vi "Stage Motor Test.vi"() -> ()   [LabVIEW 2016]
uses:
  <vilib>/Platform/TimedLoop/XDataNode/timing_clust.ctl
  <vilib>/Platform/TimedLoop/XDataNode/nitl_modes.ctl
  <vilib>/Platform/TimedLoop/XDataNode/wakeup.ctl
  <vilib>/DAQmx/write.llb/DAQmx Write (Analog 1D DBL NChan 1Samp).vi
  <vilib>/FPGAPlugInAG/PXI-7833R/niLvFpga_Open_PXI-7833R.vi
  <vilib>/Utility/error.llb/Error Cluster From Error Code.vi
  <vilib>/rvi/errors/niLvFpgaAdjustHostInterfaceError.vi
  <vilib>/DAQmx/create/channels.llb/DAQmx Create Channel (AO-Voltage-Basic).vi
  <vilib>/DAQmx/miscellaneous.llb/DAQmx Fill In Error Info.vi
  <vilib>/FPGAPlugInAG/PXI-7833R/niLvFpga_Reset_PXI-7833R.vi
  <vilib>/FPGAPlugInAG/PXI-7833R/niLvFpga_Close_PXI-7833R.vi
  <vilib>/Platform/TimedLoop/XDataNode/XDataNode.xnode
  <vilib>/rvi/interface/nirviOpenFPGA/nirviOpenFPGA.xnode
  FPGA Bitfiles/PhantomControlPI_FPGATarget_QuadCtr2_E2412E44.lvbitx
  IRISS_FPGA_IO.vi
  <vilib>/rvi/interface/nirviReadWriteControl/nirviReadWriteControl.xnode
  <vilib>/rvi/interface/nirviMethod/nirviMethod.xnode
  <vilib>/rvi/interface/nirviCloseFPGA/nirviCloseFPGA.xnode
  <vilib>/Platform/TimedLoop/XDataNode/XDNodeRunTimeDep.lvlib
  NiFpgaLv.dll
panel:
  out "Waveform Chart":T1(graph)
  out "Error(s) Out on Program End":errorcluster
  in  "Stage PID Cluster":T2={"Stage Z PID"={"Kp"=0.0005, "Kd"=0.001, "Ki"=0.0}, "Stage Y PID"={"Kp"=0.0003, "Kd"=0.01, "Ki"=0.0}, "Stage X PID"={"Kp"=0.0003, "Kd"=0.01, "Ki"=0.0}}
  in  "Stage cmd Posit [mm]":dbl[](array[numeric])=[12.0, 0.0, 0.0] min=0.0 max=12.0 step=0.1
  out "Stage out Posit [mm]":dbl[](array[numeric])=[12.0, 0.0, 0.0]
  in  "stop":bool
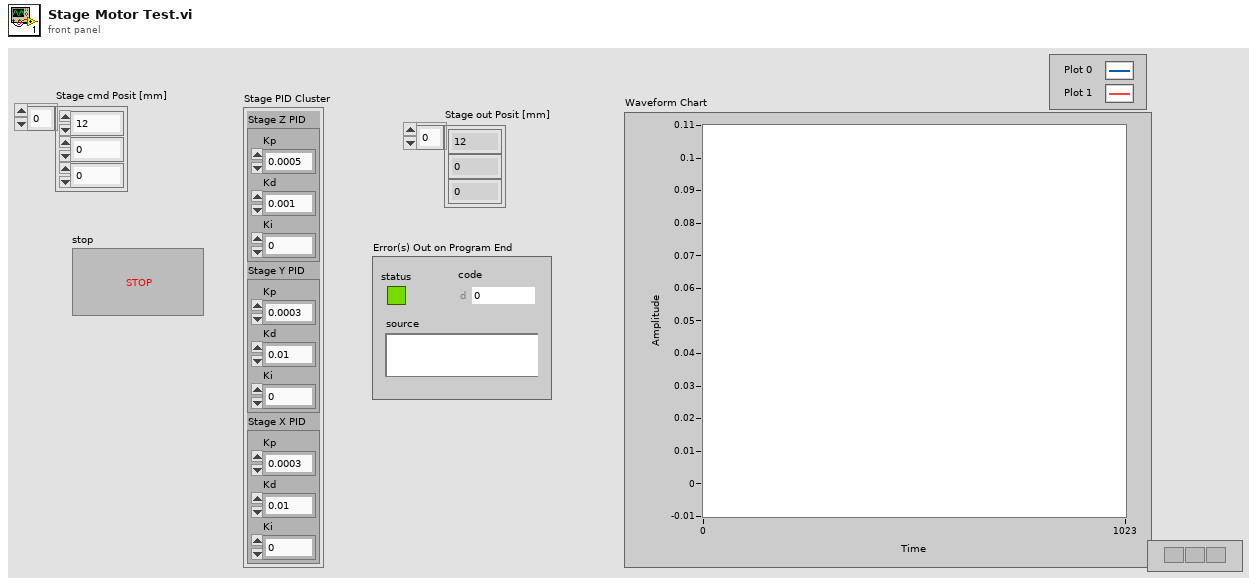
[diagram p1: front panel]
types:
  T1 = cluster{"StagePosition - X":dbl, "StagePosition - X":dbl}
  T2 = cluster{"Stage Z PID":cluster{"Kp":dbl, "Kd":dbl, "Ki":dbl}, "Stage Y PID":cluster{"Kp":dbl, "Kd":dbl, "Ki":dbl}, "Stage X PID":cluster{"Kp":dbl, "Kd":dbl, "Ki":dbl}}
  T3 = typedef "XDNodeRunTimeDep.lvlib/timing_clust.ctl" = cluster{"Expected End [f-1]":u64, "Actual End [f-1]":u64, "Finished Late? [f-1]":bool, "Expected End [i-1]":u64, "Actual End [i-1]":u64, "Finished Late? [i-1]":bool, "Expected Start [i]":u64, "Actual Start [i]":u64, "Expected Start [f]":u64, "Actual Start [f]":u64, "Source Name":string, "Structure Name":string, "Period":i64, "Deadline":i64, "Offset":i64, "Start":i64, "Priority":i32, "Timeout":i32, "Mode":T4, "Wakeup Reason":T5, "Error":errorcluster, "Source Type":string, "Secondary Source Type":string, "Global End Time":u64, "Global Start Time":u64, "Frame Duration":u64, "Iteration Duration":u64, "Assigned CPU":i32, "I/O Scan Engine Mode":u32}
  T4 = typedef "XDNodeRunTimeDep.lvlib/nitl_modes.ctl" = enum32{"No Change", "Process missed periods, maintain original phase", "Discard missed periods, maintain original phase", "Process missed periods, ignore original phase", "Discard missed periods, ignore original phase"}
  T5 = typedef "XDNodeRunTimeDep.lvlib/wakeup.ctl" = enum32{"Normal", "Aborted", "Asynchronous wakeup", "Timing source error", "Timed loop error", "Timeout"}
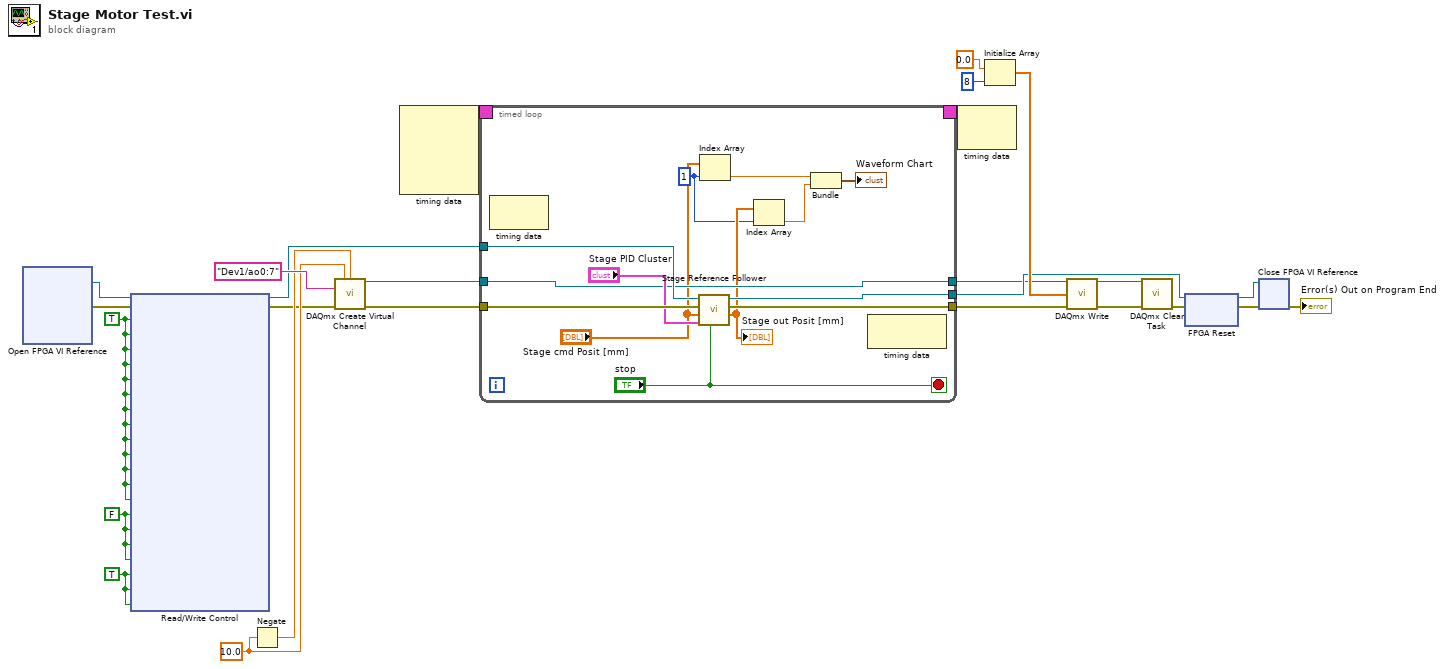
[diagram p0: block diagram]
diagram:
  w18 = 10.0
  w23 = TRUE ("Conn0/DIO12 Button 1")
  w22 = FALSE ("Reset")
  w24 = TRUE ("Reset")
  n1 = xnode "Open FPGA VI Reference"() -> ("FPGA VI Reference Out"=w21:refnum<k20>, "error out"=w20:errorcluster)  [unwired: 2 in]
  n2 = xnode "Read/Write Control"("FPGA VI Reference In"=w21, "error in"=w20, "Reset 1"=w24, "Reset 3"=w24, "Reset 9"=w24, "Reset 10"=w24, "Reset 11"=w24, "Reset 12"=w24, "Reset 13"=w24, "Reset 14"=w24, "Reset 15"=w24, "Reset 16"=w24, "Reset 17"=w24, "Reset C1-1"=w24, "Reset C1-4"=w24, "INHB X"=w22, "INHB Y"=w22, "INHB Z"=w22, "INHB OCT Mot"=w22, "Conn0/DIO12 Button 1"=w23, "Conn0/DIO13 Button 2"=w23, "Conn0/DIO15 Button 4"=w23) -> ("FPGA VI Reference Out"=w14:refnum<k20>, "error out"=w16:errorcluster)
  n3 = Negate(x=w18) -> (-x=w17:dbl)
  n4 = call-poly <vilib>:"DAQmx Create Virtual Channel.vi"("maximum value"=w18, "minimum value"=w17, "physical channels"="Dev1/ao0:7", "error in"=w16) -> ("task out"=w1:refnum<k21>, "error out"=w15:errorcluster)  [unwired: 10 in]
  n5 = node-c288() -> (w26:T3)  [unwired: 4 in]
  n6 = timed-loop {
    timing: w26 -> [_]
    timing-out: [_] -> w25
    tunnel: [w39] -> w4
    tunnel: w15 -> [w38]
    tunnel: w14 -> [w36]
    tunnel: [w35] -> w3
    tunnel: [w34] -> w2
    tunnel: w1 -> [w34]
    stop <- "stop" stop-if-true
    w30 = 1 ("index")
    n7 = node-c288() -> ()  [unwired: 1 in, 1 out]
    n8 = call "Stage Reference Follower.vi"("stop"="stop", "Stage PID Cluster"="Stage PID Cluster", "Stage cmd Posit [mm]"="Stage cmd Posit [mm]", "error in"=w38, "FPGA VI Reference In"=w36) -> ("Stage out Posit [mm]"=w31:dbl[], "error out"=w35:errorcluster, "FPGA VI Reference Out"=w39:refnum<k20>)  [unwired: 4 in]
    "Stage out Posit [mm]" <- w31
    n9 = Index Array(array="Stage cmd Posit [mm]", index=w30) -> (element=w27:dbl)
    n10 = Index Array(array=w31, index=w30) -> (element=w28:dbl)
    n11 = Bundle("StagePosition - X"=w27, "StagePosition - X"=w28) -> (→"Waveform Chart":T1)  [unwired: 1 in]
    n12 = node-c288() -> ()  [unwired: 1 in, 1 out]
  }
  n13 = node-c288(w25) -> ()  [unwired: 1 out]
  n14 = Initialize Array(0.0 ("element"), 8 ("dimension size")) -> (w8:dbl[])
  n15 = call-poly <vilib>:"DAQmx Write.vi"("task/channels in"=w2, "data"=w8, "error in"=w3) -> ("task out"=w7:refnum<k21>, "error out"=w6:errorcluster)  [unwired: 10 in, 1 out]
  n16 = call <vilib>:"DAQmx Clear Task.vi"("task in"=w7, "error in"=w6) -> ("error out"=w5:errorcluster)  [unwired: 13 in]
  n17 = xnode "FPGA Reset"("FPGA VI Reference In"=w4, "error in"=w5) -> ("FPGA VI Reference Out"=w13:refnum<k20>, "error out"=w12:errorcluster)
  n18 = xnode "Close FPGA VI Reference"("FPGA VI Reference In"=w13, "error in"=w12) -> ("error out"=→"Error(s) Out on Program End":errorcluster)
